vi "Commit Hardware Relay State.vi"(0 "PhysicalChannelRelay in":refnum<class "PhysicalChannelRelay.lvclass">, 5 "Session Handle in":T1, 11 "error in (no error)":errorcluster) -> (4 "PhysicalChannelRelay out":refnum<class "PhysicalChannelRelay.lvclass">, 15 "error out":errorcluster)   [LabVIEW 2015, in "SLSC Switch.lvlib" / "PhysicalChannelRelay.lvclass"]
uses:
  PhysicalChannelRelay.lvclass
  SLSC Session/Typedefs/Session Handle.ctl
  SLSC Session/SLSC Session.lvclass
  Relay Interface/Commit Buffer Action.ctl
  Relay Interface/RelayInterface.lvclass
  SLSC Switch/SLSC Switch.lvclass
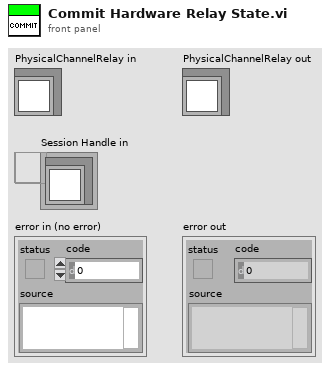
[diagram p1: front panel]
types:
  T1 = typedef "SLSC Switch.lvlib/SLSC Session.lvclass/Session Handle.ctl" = refnum<data-value>
  T2 = typedef "SLSC Switch.lvlib/RelayInterface.lvclass/Commit Buffer Action.ctl" = enum16{"Get Session Buffer", "Add Transaction", "Clear Session Buffer", "Clear All"}
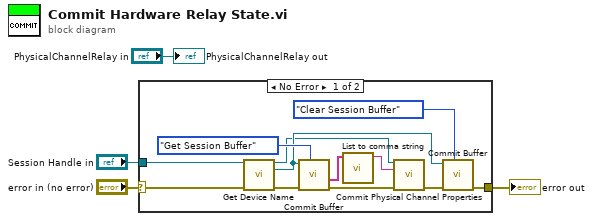
[diagram p0: block diagram]
diagram:
  n1 = case shown="No Error" "error in (no error)" {
    selector: "error in (no error)" -> [w12 w17]
    tunnel: [w10 w17] -> w2
    tunnel: "Session Handle in" -> [w14 _]
    frame No Error {
      n2 = call "Get Device Name.vi"("Session Handle in"=w14, "error in (no error)"=w12) -> ("Session Handle out"=w6:T1, "device"=w9:refnum<k21>, "error out"=w11:errorcluster)  [unwired: 11 in]
      n3 = call "Commit Buffer.vi"("Action"=Commit_Buffer_Action."Get Session Buffer", "error in (no error)"=w11, "device name in"=w9) -> ("error out"=w8:errorcluster, "Transactions"=w13:string[])  [unwired: 7 in]
      n4 = call "List to comma string.vi"("Array"=w13) -> ("String"=w5:string)  [unwired: 10 in]
      n5 = call "Commit Physical Channel Properties.vi"("Session Handle in"=w6, "physical channels"=w5, "error in (no error)"=w8) -> ("error out"=w7:errorcluster)  [unwired: 11 in, 1 out]
      n6 = call "Commit Buffer.vi"("Action"=Commit_Buffer_Action."Clear Session Buffer", "error in (no error)"=w7, "device name in"=w9) -> ("error out"=w10:errorcluster)  [unwired: 7 in, 1 out]
    }
    frame Error {
    }
  }
  "error out" <- w2
  "PhysicalChannelRelay out" <- "PhysicalChannelRelay in"
